vi "Needs Firmware Update.vi"(8 "error in (no error)":errorcluster, 11 "FirmwareRev":string) -> (0 "error out":errorcluster, 3 "Update?":bool)   [LabVIEW 2020]
doc: "This VI determines if the RT device's firmware is compatible with SystemLink Client, which means it must be higher than version 6."
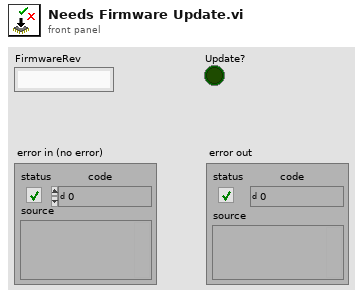
[diagram p1: front panel]
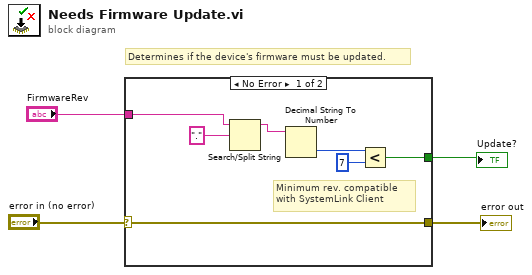
[diagram p0: block diagram]
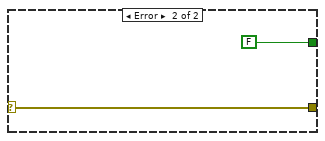
[diagram p2: hidden frame]
diagram:
  # "Determines if the device's firmware must be updated."
  n1 = case shown="No Error" "error in (no error)" {
    selector: "error in (no error)" -> [w8 w13]
    tunnel: [w8 w13] -> w3
    tunnel: [w7 FALSE] -> w2
    tunnel: "FirmwareRev" -> [w6 _]
    frame No Error {
      # "Minimum rev. compatible\nwith SystemLink Client"
      n2 = Search/Split String(string=w6, search string/char (-)="." ("regular expression")) -> (substring before match=w5:string)  [unwired: 1 in, 2 out]
      n3 = Decimal String To Number(string=w5) -> (number=w10:i32)  [unwired: 2 in, 1 out]
      n4 = Less?(x=w10, y=7) -> (x < y?=w7:bool)
    }
    frame Error {
    }
  }
  "error out" <- w3
  "Update?" <- w2
